vi "Rx Begin.vi"(8 "error in (no error)":errorcluster, 11 "Framework in":refnum<class "Framework.lvclass">) -> (0 "error out":errorcluster, 3 "Framework out":refnum<class "Framework.lvclass">)   [LabVIEW 2017, in "DSF Core.lvlib" / "Framework.lvclass"]
uses:
  Framework.lvclass
  Framework.lvclass/Framework.ctl
  Performance/Performance.lvclass/Performance.ctl
  Performance/Performance.lvclass
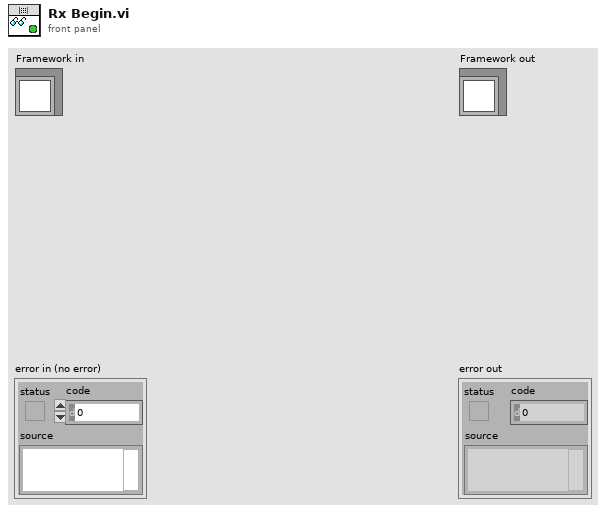
[diagram p1: front panel]
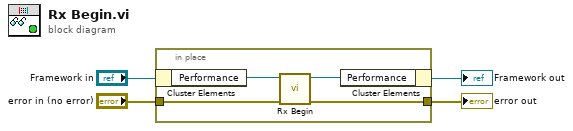
[diagram p0: block diagram]
diagram:
  n1 = in-place {
    in-place-border: "error in (no error)" -> [w6]
    in-place-border: [w5] -> w1
    n2 = in-place-cluster #1("Framework in") -> ("Performance"=w8:refnum<class "Performance.lvclass">)
    n3 = call "Rx Begin.vi"("error in (no error)"=w6, "Performance in"=w8) -> ("error out"=w5:errorcluster, "Performance out"=w7:refnum<class "Performance.lvclass">)  [unwired: 8 in]
    n4 = in-place-cluster #1("Performance"=w7) -> (→"Framework out":refnum<class "Framework.lvclass">)
  }
  "error out" <- w1
